vi "0036-Sub_calc_HDC1080.vi"(8 "humi":u8[](array[numeric]), 10 "temp":u8[](array[numeric])) -> (1 "humi":dbl, 3 "temp":dbl)   [LabVIEW 2014]
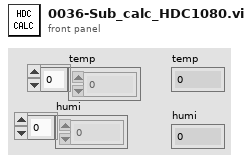
[diagram p1: front panel]
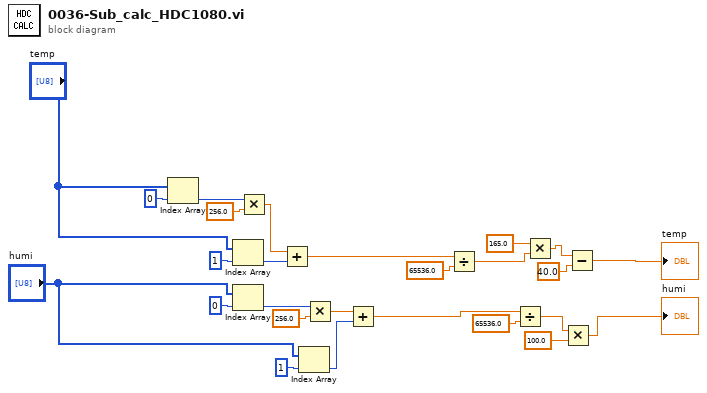
[diagram p0: block diagram]
diagram:
  n1 = Index Array(array="temp", index=0 ("指標")) -> (element=w14:u8)
  n2 = Index Array(array="temp", index=1 ("指標")) -> (element=w17:u8)
  n3 = Index Array(array="humi", index=0 ("指標")) -> (element=w24:u8)
  n4 = Multiply(x=w14, y=256.0) -> (x*y=w16:dbl)
  n5 = Add(x=w16, y=w17) -> (x+y=w10:dbl)
  n6 = Index Array(array="humi", index=1 ("指標")) -> (element=w25:u8)
  n7 = Multiply(x=w24, y=256.0) -> (x*y=w22:dbl)
  n8 = Add(x=w22, y=w25) -> (x+y=w4:dbl)
  n9 = Divide(x=w10, y=65536.0) -> (x/y=w9:dbl)
  n10 = Divide(x=w4, y=65536.0) -> (x/y=w3:dbl)
  n11 = Multiply(x=165.0, y=w9) -> (x*y=w6:dbl)
  n12 = Multiply(x=w3, y=100.0) -> (x*y=→"humi":dbl)
  n13 = Subtract(x=w6, y=40.0 ("x")) -> (x-y=→"temp":dbl)
